vi "CloseAppRefInCluster.vi"(1 "Cluster":cluster{"App Refnum":refnum<vi>}) -> (0 "error out":errorcluster)   [LabVIEW 2010]
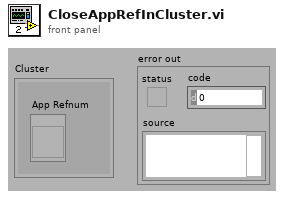
[diagram p1: front panel]
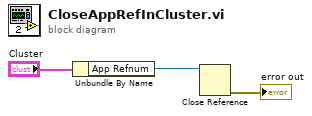
[diagram p0: block diagram]
diagram:
  n1 = Unbundle By Name("Cluster") -> ("App Refnum"=w1:refnum<vi>)
  n2 = Close Reference(reference=w1) -> (error out=→"error out":errorcluster)  [unwired: 1 in]
